vi "流程参数写入.vi"(7 "是否启用通讯通知":bool, 8 "error in (no error)":errorcluster, 10 "参数":T1, 11 "Slave ID":T2) -> (0 "error out":errorcluster)   [LabVIEW 2016, in "质控单元V1.lvlib"]
uses:
  <vilib>/Plasmionique/MB Master/MB_Master/MB_Master.lvclass
  <vilib>/Plasmionique/MB Master/MB Master.lvlib
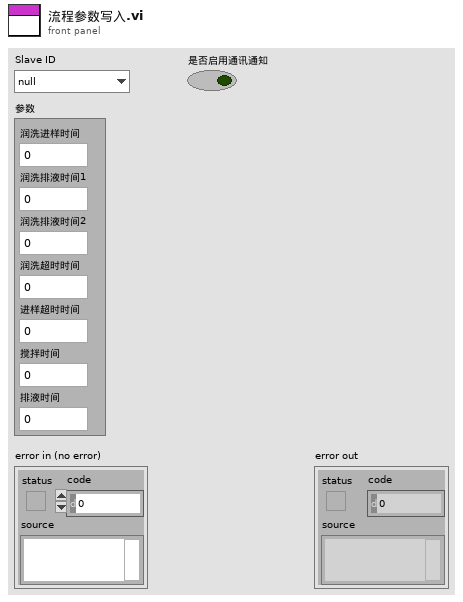
[diagram p1: front panel]
types:
  T1 = cluster{"润洗进样时间":sgl, "润洗排液时间1":sgl, "润洗排液时间2":sgl, "润洗超时时间":sgl, "进样超时时间":sgl, "搅拌时间":sgl, "排液时间":sgl}
  T2 = typedef "质控单元V1.lvlib/质控slave id.ctl" = enum16{"null", "氨氮", "总磷", "CODMn", "CODCr", "总氮"}
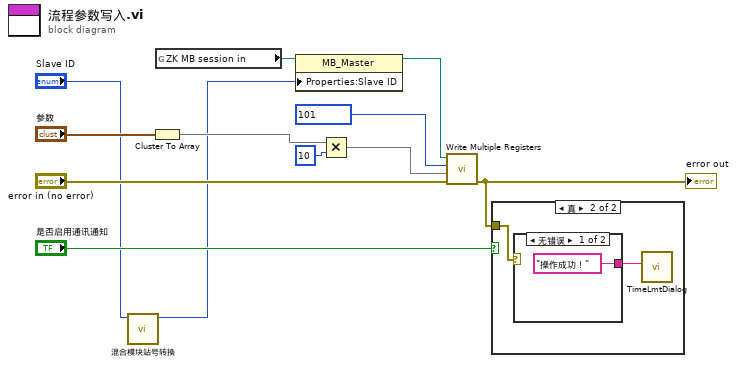
[diagram p0: block diagram]
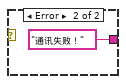
[diagram p3: hidden frame]
diagram:
  n1 = call "混合模块站号转换.vi"("Slave ID输入"="Slave ID") -> ("Slave ID输出"=w1:T2)  [unwired: 10 in]
  n2 = Cluster To Array(cluster="参数") -> (array=w5:sgl[])
  n3 = global read "ZK非断电保存全局变量.vi" "ZK MB session in"() -> (w11:refnum<class "MB_Master.lvclass">)
  n4 = property class="MB_Master"(reference=w11, "Properties:Slave ID"=w1) -> (reference out=w9:refnum<class "MB_Master.lvclass">)  [unwired: 1 in, 1 out]
  n5 = Multiply(x=w5, y=10) -> (x*y=w3:sgl[])
  n6 = call <vilib>:"Write Multiple Registers.vi"("error in (no error)"="error in (no error)", "values"=w3, "starting address"=u16 101, "MB session in"=w9) -> ("error out"=w7:errorcluster)  [unwired: 6 in, 1 out]
  "error out" <- w7
  n7 = case shown="真" "是否启用通讯通知" {
    tunnel: w7 -> [_ w14]
    frame False {
    }
    frame True {
      n8 = case shown="无错误" w14 {
        tunnel: ["操作成功！" "通讯失败！"] -> w13
        frame No Error {
        }
        frame Error {
        }
      }
      n9 = call "TimeLmtDialog.vi"("Infoin"=w13) -> ()  [unwired: 11 in]
    }
  }
